vi "FAMM_Write Gserver-Queue.vi"(8 "error in (no error)":errorcluster, 10 "Gserver-Queue":refnum<queue>, 11 "FAMM in":refnum<class "FAMM.lvclass">) -> (0 "error out":errorcluster, 3 "FAMM out":refnum<class "FAMM.lvclass">)   [LabVIEW 2020, in "FAMM.lvclass"]
uses:
  FAMM.lvclass
  Gserver/controls/Typedef_Gviewer-Query.ctl
  Gserver/controls/Typedef_QueryType.ctl
  FAMM.lvclass/FAMM.ctl
  Gserver/Gserver.lvclass
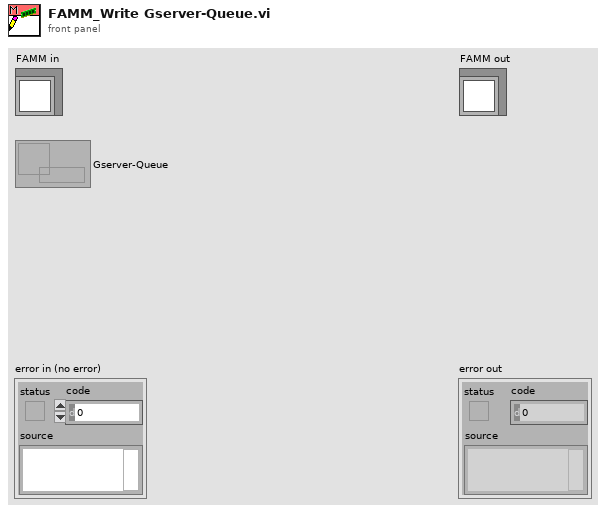
[diagram p1: front panel]
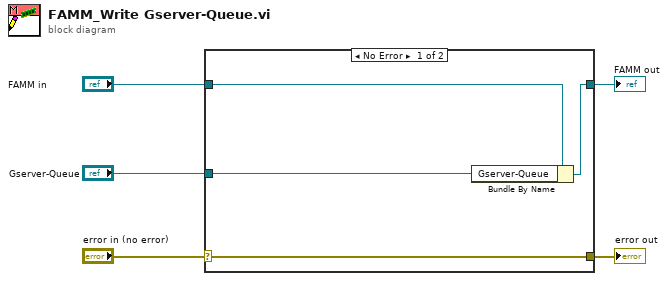
[diagram p0: block diagram]
diagram:
  n1 = case shown="No Error" "error in (no error)" {
    selector: "error in (no error)" -> [w9 w10]
    tunnel: [w9 w10] -> w4
    tunnel: [w7 w11] -> w2
    tunnel: "FAMM in" -> [w8 w11]
    tunnel: "Gserver-Queue" -> [w6 _]
    frame No Error {
      n2 = Bundle By Name(cluster=w8, "Gserver-Queue"=w6) -> (w7:refnum<class "FAMM.lvclass">)
    }
    frame Error {
    }
  }
  "error out" <- w4
  "FAMM out" <- w2
